vi "Stop Discovery.vi"   [LabVIEW 2020, in "epl-network.lvlib"]
uses:
  epl-network.lvlib
  afc993c7-4e33-4e74-80a4-61b5b983949b.vi
types:
  T1 = typedef "epl-network.lvlib/Discovery FGV.ctl" = cluster{"loops":refnum<vi>, "stop":refnum<notifier>, "events":cluster{"DiscoveredHost":refnum<user-event>, "ExpiredHost":refnum<user-event>}}
  T2 = cluster{"DiscoveredHost":refnum<user-event>, "ExpiredHost":refnum<user-event>}
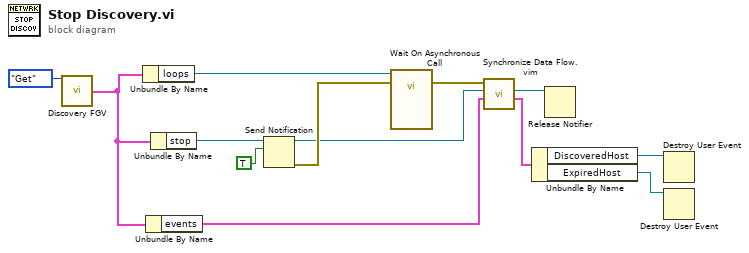
[diagram p0: block diagram]
diagram:
  n1 = call "Discovery FGV.vi"("action"=enum16{"Initialize", "Get"}."Get") -> ("data out"=w5:T1)  [unwired: 14 in]
  n2 = Unbundle By Name(w5) -> ("loops"=w11:refnum<vi>)
  n3 = Unbundle By Name(w5) -> ("events"=w4:T2)
  n4 = Unbundle By Name(w5) -> ("stop"=w8:refnum<notifier>)
  n5 = Send Notification(notification=TRUE, notifier=w8) -> (notifier out=w7:refnum<notifier>, error out=w10:errorcluster)  [unwired: 1 in]
  n6 = call-by-ref "Wait On Asynchronous Call"(reference=w11, error in=w10) -> (error out=w9:errorcluster)  [unwired: 15 in, 2 out]
  n7 = call "Synchronize Data Flow.vim"("input 3"=w4, "input 2"=w7, "input 1"=w9) -> ("output 3"=w3:T2, "output 2"=w6:refnum<notifier>)  [unwired: 1 in, 2 out]
  n8 = Unbundle By Name(w3) -> ("DiscoveredHost"=w2:refnum<user-event>, "ExpiredHost"=w1:refnum<user-event>)
  n9 = Release Notifier(notifier=w6) -> ()  [unwired: 2 in, 3 out]
  n10 = Destroy User Event(user event=w2) -> ()  [unwired: 1 in, 1 out]
  n11 = Destroy User Event(user event=w1) -> ()  [unwired: 1 in, 1 out]
